vi "plc_registers.vi"() -> ()   [LabVIEW 2023]
panel:
  in  "Array":T1(array[cluster])=[{"Name"="Rotate_CMD", "Address"=0, "Data Type"=enum."Int", "Reg Type"=enum."Input"}, {"Name"="Termex_CMD", "Address"=1, "Data Type"=enum."Int", "Reg Type"=enum."Input"}, {"Name"="Mix_CMD", "Address"=2, "Data Type"=enum."Int", "Reg Type"=enum."Input"}, {"Name"="Rotate_SP_Angle_Init", "Address"=3, "Data Type"=enum."Int", "Reg Type"=enum."Input"}, {"Name"="Rotate_SP_Angle_End", "Address"=4, "Data Type"=enum."Int", "Reg Type"=enum."Input"}, {"Name"="Rotate_SP_Timeout", "Address"=5, "Data Type"=enum."Int", "Reg Type"=enum."Input"}, {"Name"="Rotate_SP_Speed", "Address"=6, "Data Type"=enum."Int", "Reg Type"=enum."Input"}, {"Name"="Reserved", "Address"=7, "Data Type"=enum."Int", "Reg Type"=enum."Input"}, {"Name"="T_SP", "Address"=8, "Data Type"=enum."Float", "Reg Type"=enum."Input"}, {"Name"="KP", "Address"=10, "Data Type"=enum."Float", "Reg Type"=enum."Input"}, {"Name"="TN", "Address"=12, "Data Type"=enum."Float", "Reg Type"=enum."Input"}, {"Name"="Mix_SP", "Address"=14, "Data Type"=enum."Int", "Reg Type"=enum."Input"}, {"Name"="Reserved", "Address"=15, "Data Type"=enum."Int", "Reg Type"=enum."Input"}, {"Name"="Reserved", "Address"=16, "Data Type"=enum."Int", "Reg Type"=enum."Input"}, {"Name"="Reserved", "Address"=17, "Data Type"=enum."Int", "Reg Type"=enum."Input"}, {"Name"="Reserved", "Address"=18, "Data Type"=enum."Int", "Reg Type"=enum."Input"}]
  out "Output Map":T2(c390)
  out "Array 2":T1(array[cluster])=[{"Name"="Rotate_IND", "Address"=0, "Data Type"=enum."Int", "Reg Type"=enum."Input"}, {"Name"="Termex_IND", "Address"=1, "Data Type"=enum."Int", "Reg Type"=enum."Input"}, {"Name"="Mix_IND", "Address"=2, "Data Type"=enum."Int", "Reg Type"=enum."Input"}, {"Name"="Rotate_PV_Angle_Init", "Address"=3, "Data Type"=enum."Int", "Reg Type"=enum."Input"}, {"Name"="Rotate_PV_Angle_End", "Address"=4, "Data Type"=enum."Int", "Reg Type"=enum."Input"}, {"Name"="Rotate_PV_Timeout", "Address"=5, "Data Type"=enum."Int", "Reg Type"=enum."Input"}, {"Name"="Rotate_PV_Speed", "Address"=6, "Data Type"=enum."Int", "Reg Type"=enum."Input"}, {"Name"="Rotate_PV_Time", "Address"=7, "Data Type"=enum."Int", "Reg Type"=enum."Input"}, {"Name"="Rotate_PV_Angle", "Address"=8, "Data Type"=enum."Int", "Reg Type"=enum."Input"}, {"Name"="Termex_PV_In", "Address"=9, "Data Type"=enum."Float", "Reg Type"=enum."Input"}, {"Name"="Termex_PV_Out", "Address"=11, "Data Type"=enum."Float", "Reg Type"=enum."Input"}, {"Name"="Termex_SP", "Address"=13, "Data Type"=enum."Float", "Reg Type"=enum."Input"}, {"Name"="Termex_KP", "Address"=15, "Data Type"=enum."Float", "Reg Type"=enum."Input"}, {"Name"="Termex_TN", "Address"=17, "Data Type"=enum."Float", "Reg Type"=enum."Input"}, {"Name"="MIX_PV", "Address"=19, "Data Type"=enum."Int", "Reg Type"=enum."Input"}, {"Name"="P_PV", "Address"=20, "Data Type"=enum."Float", "Reg Type"=enum."Input"}, {"Name"="MM_PV", "Address"=22, "Data Type"=enum."Float", "Reg Type"=enum."Input"}]
  out "IND":T3 {"Rotate_IND" items=["стоп", "Качалка Режим Авто", "Качалка Режим Ручной"]; "Termex_IND" items=["Термостат старт"=1, "Термостат стоп"=0]; "Mix_IND" items=["Мешалка движение вперёд"=1, "Мешалка движение назад"=2, "Мешалка стоп"=0]}
  in  "CMD":T4 {"Mix_CMD" items=["Мешалка движение вперёд"=1, "Мешалка движение назад"=2, "Мешалка стоп"=9]; "Termex_CMD" items=["Термостат старт"=1, "Термостат стоп"=9]; "Rotate_CMD" items=["Качалка Дом"=1, "Качалка Режим Авто - Старт"=2, "Качалка Режим Ручной - Старт"=3, "Качалка Стоп"=9]}
  in  "all rows":string[][](array[string])=[["Control", "Адрес", "CMD", "Комментарий", "", "Indication", "Адрес", "ÑMD", "Комментарий"], ["Rotate_CMD", "0", "1", "(*Качалка Дом*)", "", "Rotate_IND", "0", "0", "стоп"], ["", "0", "2", "(*Качалка Режим Авто - Старт*)", "", "", "0", "1", "(*Качалка Режим Авто*)"], ["", "0", "3", "(*Качалка Режим Ручной - Старт*)", "", "", "0", "2", "(*Качалка Режим Ручной*)"], ["", "0", "9", "(*Качалка Стоп*)", "", "", "", "", ""], ["Termex_CMD", "1", "1", "(*Термостат старт*)", "", "Termex_IND", "1", "1", "(*Термостат старт*)"], ["", "1", "9", "(*Термостат стоп*)", "", "", "1", "0", "(*Термостат стоп*)"], ["Mix_CMD", "2", "1", "(*Мешалка движение вперёд*)", "", "Mix_IND", "2", "1", "(*Мешалка движение вперёд*)"], ["", "2", "2", "(*Мешалка движение назад*)", "", "", "2", "2", "(*Мешалка движение назад*)"], ["", "2", "9", "(*Мешалка стоп*)", "", "", "2", "0", "(*Мешалка стоп*)"], ["Rotate_SP_Angle_Init", "3", "", "(*Качалка начальный угол*)", "", "Rotate_PV_Angle_Init", "3", "", "(*Качалка заданный начальный угол*)"], ["Rotate_SP_Angle_End", "4", "", "(*Качалка конечный угол*)", "", "Rotate_PV_Angle_End", "4", "", "(*Качалка заданный конечный угол*)"], ["Rotate_SP_Timeout", "5", "", "(*Качалка время паузы*)", "", "Rotate_PV_Timeout", "5", "", "(*Качалка заданное время паузы*)"], ["Rotate_SP_Speed", "6", "", "(*Качалка скорость вращения*)", "", "Rotate_PV_Speed", "6", "", "(*Качалка заданная скорость вращения*)"], ["Reserved", "7", "", "", "", "Rotate_PV_Time", "7", "", "(*Качалка отсчитанное время паузы*)"], ["T_SP[0]", "8", "", "(*Термостат уставка 1 байт*)", "", "Rotate_PV_Angle", "8", "", "(*Качалка текущий угол*)"], ["T_SP[1]", "9", "", "(*Термостат уставка 2 байт*)", "", "Termex_PV_In[0]", "9", "", "(*Термостат текущая внутр. Т 1 байт*)"], ["KP[0]", "10", "", "(*Термостат КР 1 байт*)", "", "Termex_PV_In[1]", "10", "", "(*Термостат текущая внутр. Т 2 байт*)"], ["KP[1]", "11", "", "(*Термостат КР 2 байт*)", "", "Termex_PV_Out[0]", "11", "", "(*Термостат текущая внеш. Т 1 байт*)"], ["TN[0]", "12", "", "(*Термостат TN 1 байт*)", "", "Termex_PV_Out[1]", "12", "", "(*Термостат текущая внеш. Т 2 байт*)"], ["TN[1]", "13", "", "(*Термостат TN 2 байт*)", "", "Termex_SP[0]", "13", "", "(*Термостат текущая уставка 1 байт*)"], ["Mix_SP", "14", "", "(*Мешалка задание*)", "", "Termex_SP[1]", "14", "", "(*Термостат текущая уставка 2 байт*)"], ["Reserved", "15", "", "", "", "Termex_KP[0]", "15", "", "(*Термостат текущий KP 1 байт*)"], ["Reserved", "16", "", "", "", "Termex_KP[1]", "16", "", "(*Термостат текущий KP 2 байт*)"], ["Reserved", "17", "", "", "", "Termex_TN[0]", "17", "", "(*Термостат текущий TN 1 байт*)"], ["Reserved", "18", "", "", "", "Termex_TN[1]", "18", "", "(*Термостат текущий TN 2 байт*)"], ["", "", "", "", "", "MIX_PV", "19", "", "(*Мешалка текущая скорость*)"], ["", "", "", "", "", "P_PV[0]", "20", "", "(*Давление 1 байт*)"], ["", "", "", "", "", "P_PV[1]", "21", "", "(*Давление 2 байт*)"], ["", "", "", "", "", "MM_PV[0]", "22", "", "(*Показания линейки 1 байт*)"], ["", "", "", "", "", "MM_PV[1]", "23", "", "(*Показания линейки 2 байт*)"], ["", "", "", "", "", "", "", "", ""], ["", "", "", "", "", "", "", "", ""], ["", "", "", "", "", "", "", "", ""], ["", "", "", "", "", "", "", "", ""], ["", "", "", "", "", "", "", "", ""], ["", "", "", "", "", "", "", "", ""], ["", "", "", "", "", "", "", "", ""], ["", "", "", "", "", "", "", "", ""], ["", "", "", "", "", "", "", "", ""], ["", "", "", "", "", "", "", "", ""], ["", "", "", "", "", "", "", "", ""], ["", "", "", "", "", "", "", "", ""], ["", "", "", "", "", "", "", "", ""], ["", "", "", "", "", "", "", "", ""]]
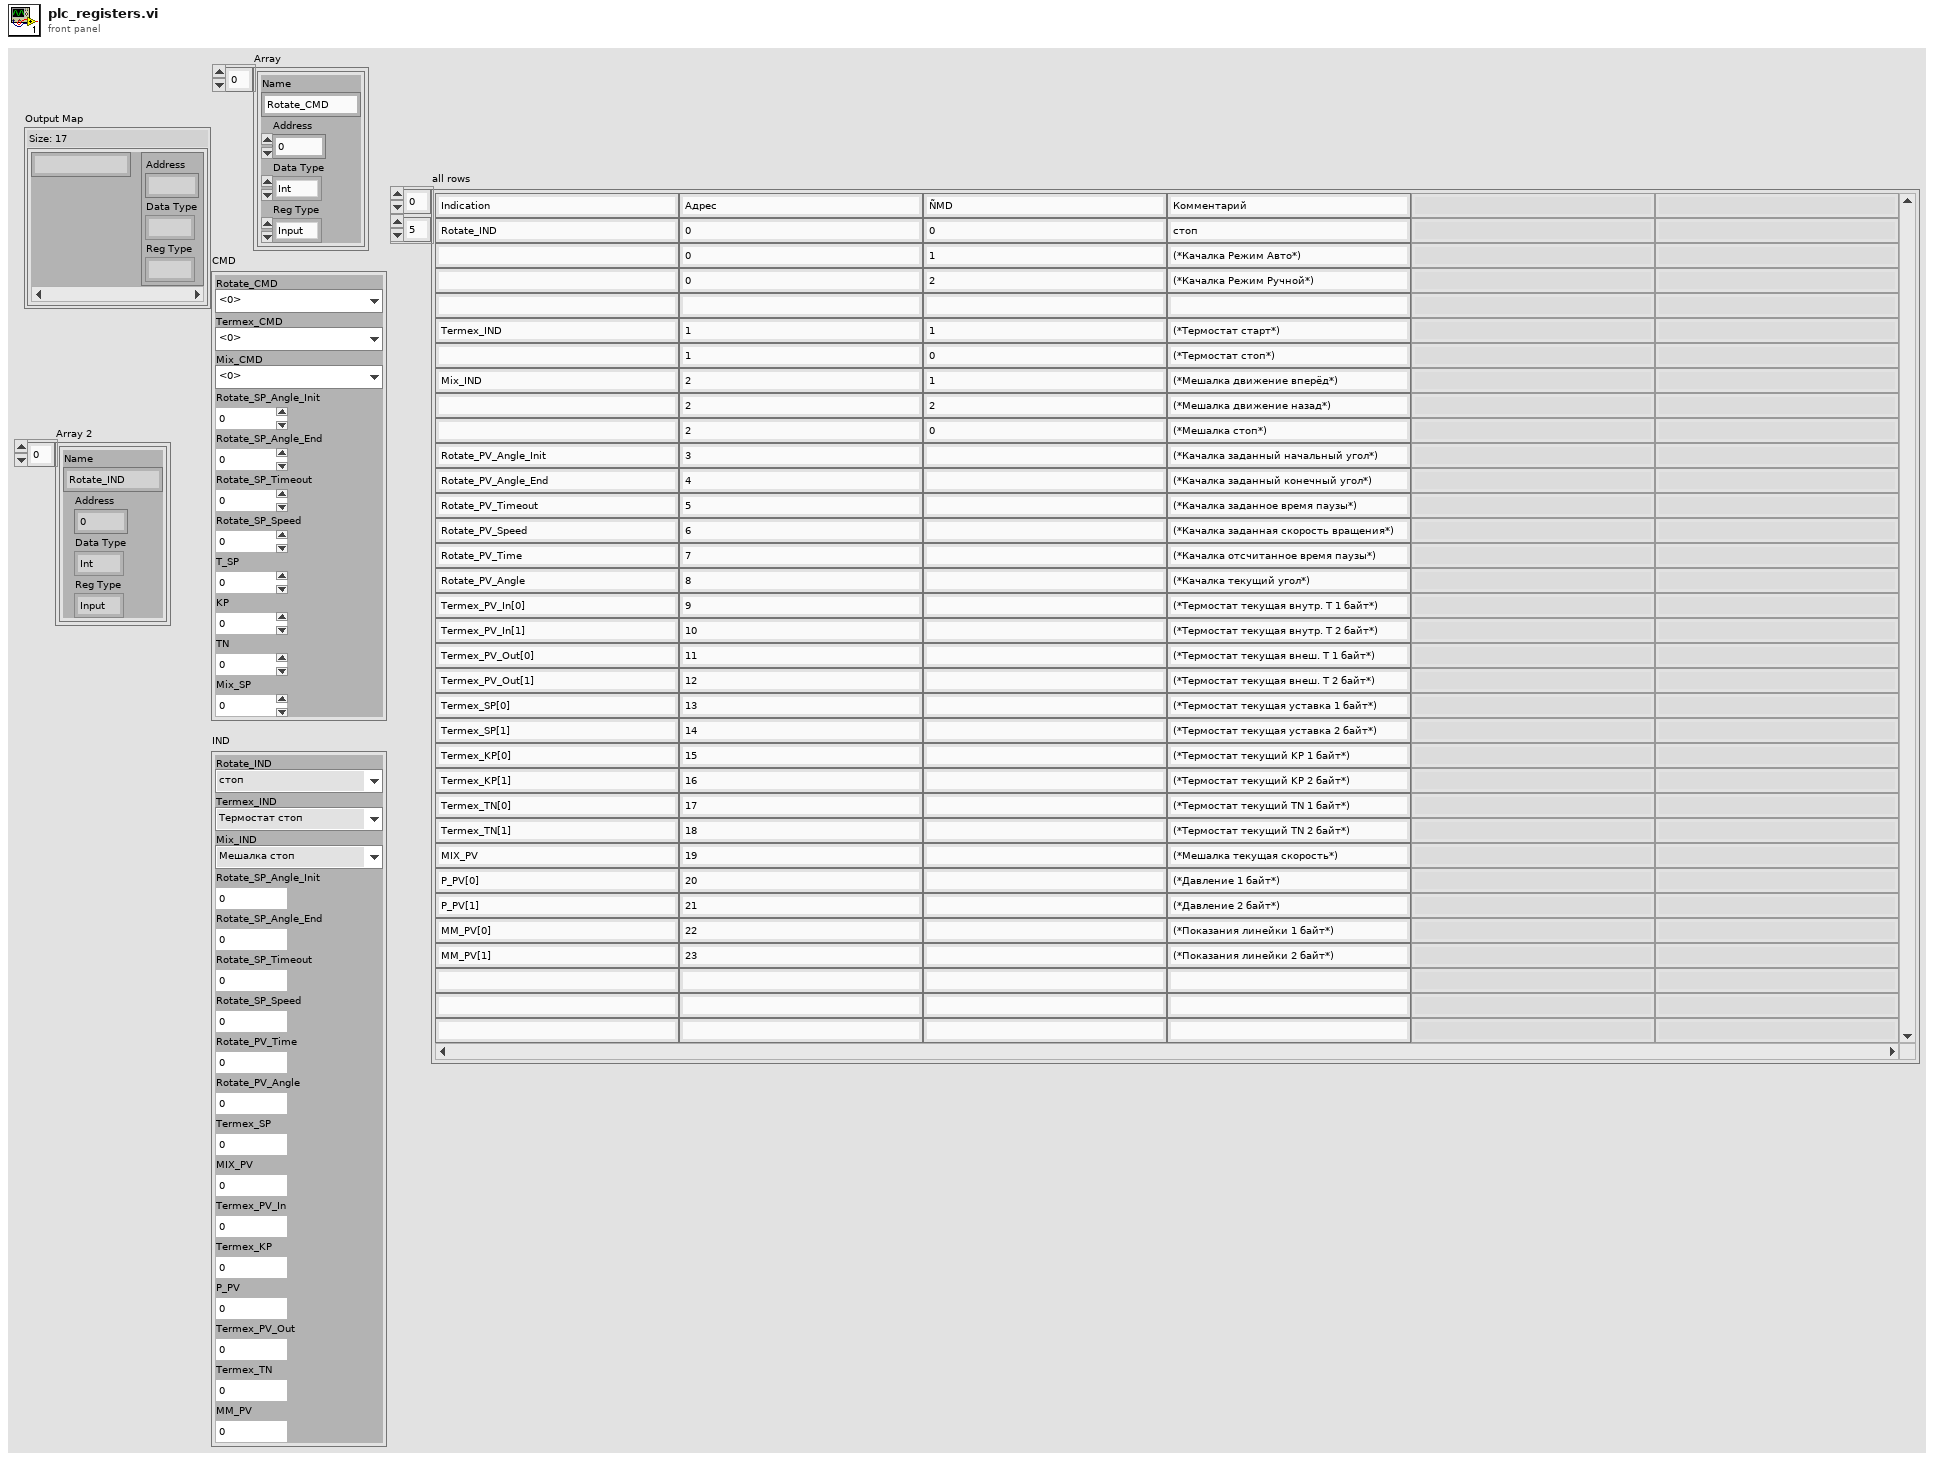
[diagram p1: front panel]
types:
  T1 = cluster{"Name":string, "Address":i32, "Data Type":enum16{"Int", "Float"}, "Reg Type":enum16{"Holding", "Input", "Coil"}}[]
  T2 = map{string, cluster{"Address":i32, "Data Type":enum16{"Int", "Float"}, "Reg Type":enum16{"Holding", "Input", "Coil"}}}
  T3 = cluster{"Rotate_IND":u16, "Termex_IND":u16, "Mix_IND":u16, "Rotate_SP_Angle_Init":u16, "Rotate_SP_Angle_End":u16, "Rotate_SP_Timeout":u16, "Rotate_SP_Speed":u16, "Rotate_PV_Time":u16, "Rotate_PV_Angle":u16, "Termex_SP":sgl, "MIX_PV":u16, "Termex_PV_In":sgl, "Termex_KP":sgl, "P_PV":sgl, "Termex_PV_Out":sgl, "Termex_TN":sgl, "MM_PV":sgl}
  T4 = cluster{"Rotate_CMD":u16, "Termex_CMD":u16, "Mix_CMD":u16, "Rotate_SP_Angle_Init":u16, "Rotate_SP_Angle_End":u16, "Rotate_SP_Timeout":u16, "Rotate_SP_Speed":u16, "T_SP":sgl, "KP":sgl, "TN":sgl, "Mix_SP":u16}
  T5 = cluster{"Name":string, "Address":i32, "Data Type":enum16{"Int", "Float"}, "Reg Type":enum16{"Holding", "Input", "Coil"}}
  T6 = cluster{"Address":i32, "Data Type":enum16{"Int", "Float"}, "Reg Type":enum16{"Holding", "Input", "Coil"}}
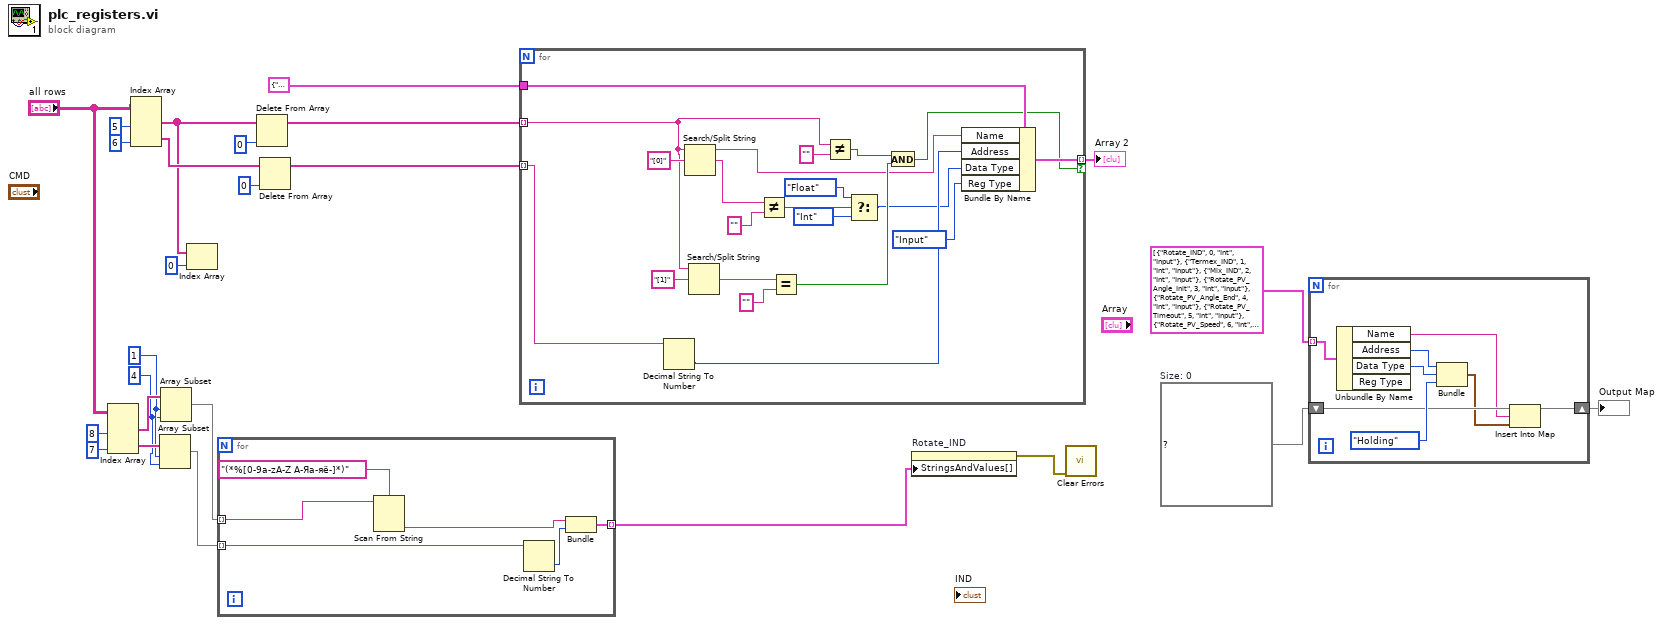
[diagram p0: block diagram]
diagram:
  w3 = T2 {}  # Size: 0
  w9 = 4 ("length")
  w10 = 1 ("index")
  n1 = Index Array(array="all rows", index (col) #1=8 ("disabled index (col)"), index (col) #2=7 ("index (col)")) -> (element #1=w12:string[], element #2=w11:string[])  [unwired: 2 in]
  n2 = Index Array(array="all rows", index (col) #1=5 ("disabled index (col)"), index (col) #2=6 ("index (col)")) -> (element #1=w15:string[], element #2=w22:string[])  [unwired: 2 in]
  n3 = Array Subset(array=w11, index=w10, length=w9) -> (w7:string[])
  n4 = Array Subset(array=w12, index=w10, length=w9) -> (w8:string[])
  n5 = Index Array(array=w15, index=0) -> ()  [unwired: 1 out]
  n6 = for {
    tunnel: w8 -> [w28] mode=indexing
    tunnel: w7 -> [w31] mode=indexing
    tunnel: [w30] -> w6 mode=indexing
    n7 = Scan From String(format string="(*%[0-9a-zA-Z А-Яа-яё-]*)", input string=w28) -> (output 1=w26:string)  [unwired: 3 in, 3 out]
    n8 = Decimal String To Number(string=w31) -> (number=w29:i32)  [unwired: 2 in, 1 out]
    n9 = Bundle(w26, w29) -> (w30:cluster{string, i32})  [unwired: 1 in]
  }
  n10 = Delete From Array(array=w15, index=0) -> (array with subset deleted=w20:string[])  [unwired: 1 in, 1 out]
  n11 = Delete From Array(array=w22, index=0) -> (array with subset deleted=w19:string[])  [unwired: 1 in, 1 out]
  n12 = for {
    tunnel: w20 -> [w32] mode=indexing
    tunnel: w19 -> [w37] mode=indexing
    tunnel: T5 {"Name"="", "Address"=0, "Data Type"=enum."Int", "Reg Type"=enum."Holding"} -> [w41]
    tunnel: [w40] -> w4 mode=indexing if=w39
    n13 = Decimal String To Number(string=w37) -> (number=w35:i32)  [unwired: 2 in, 1 out]
    n14 = Search/Split String(string=w32, search string/char (-)="[0]" ("input string")) -> (substring before match=w38:string, match + rest of string=w43:string)  [unwired: 1 in, 1 out]
    n15 = Search/Split String(string=w32, search string/char (-)="[1]" ("input string")) -> (match + rest of string=w44:string)  [unwired: 1 in, 2 out]
    n16 = Not Equal?(x=w43, y="") -> (x != y?=w49:bool)
    n17 = Equal?(x=w44, y="") -> (x = y?=w42:bool)
    n18 = Not Equal?(x=w32, y="") -> (x != y?=w46:bool)
    n19 = Select(t=enum16{"Int", "Float"}."Float", s=w49, f=enum16{"Int", "Float"}."Int") -> (s? t:f=w34:enum16{"Int", "Float"})
    n20 = And(x=w46, y=w42) -> (x .and. y?=w39:bool)
    n21 = Bundle By Name(cluster=w41, "Name"=w38, "Address"=w35, "Data Type"=w34, "Reg Type"=enum16{"Holding", "Input", "Coil"}."Input") -> (w40:T5)
  }
  "Array 2" <- w4
  n22 = property on="Rotate_IND" class="Ring (strict)"("StringsAndValues[]"=w6) -> (error out=w5:errorcluster)  [unwired: 2 in, 1 out]
  n23 = call <vilib>:"Clear Errors.vi"("error in (no error)"=w5) -> ()  [unwired: 5 in, 2 out]
  n24 = for {
    tunnel: T1 [{"Name"="Rotate_IND", "Address"=0, "Data Type"=enum."Int", "Reg Type"=enum."Input"}, {"Name"="Termex_IND", "Address"=1, "Data Type"=enum."Int", "Reg Type"=enum."Input"}, {"Name"="Mix_IND", "Address"=2, "Data Type"=enum."Int", "Reg Type"=enum."Input"}, {"Name"="Rotate_PV_Angle_Init", "Address"=3, "Data Type"=enum."Int", "Reg Type"=enum."Input"}, {"Name"="Rotate_PV_Angle_End", "Address"=4, "Data Type"=enum."Int", "Reg Type"=enum."Input"}, {"Name"="Rotate_PV_Timeout", "Address"=5, "Data Type"=enum."Int", "Reg Type"=enum."Input"}, {"Name"="Rotate_PV_Speed", "Address"=6, "Data Type"=enum."Int", "Reg Type"=enum."Input"}, {"Name"="Rotate_PV_Time", "Address"=7, "Data Type"=enum."Int", "Reg Type"=enum."Input"}, {"Name"="Rotate_PV_Angle", "Address"=8, "Data Type"=enum."Int", "Reg Type"=enum."Input"}, {"Name"="Termex_PV_In", "Address"=9, "Data Type"=enum."Float", "Reg Type"=enum."Input"}, {"Name"="Termex_PV_Out", "Address"=11, "Data Type"=enum."Float", "Reg Type"=enum."Input"}, {"Name"="Termex_SP", "Address"=13, "Data Type"=enum."Float", "Reg Type"=enum."Input"}, {"Name"="Termex_KP", "Address"=15, "Data Type"=enum."Float", "Reg Type"=enum."Input"}, {"Name"="Termex_TN", "Address"=17, "Data Type"=enum."Float", "Reg Type"=enum."Input"}, {"Name"="MIX_PV", "Address"=19, "Data Type"=enum."Int", "Reg Type"=enum."Input"}, {"Name"="P_PV", "Address"=20, "Data Type"=enum."Float", "Reg Type"=enum."Input"}, {"Name"="MM_PV", "Address"=22, "Data Type"=enum."Float", "Reg Type"=enum."Input"}] ("Array 2") -> [w60] mode=indexing
    shift-right: [w55] -> w2
    shift-left: w3 -> [w56]
    n25 = Unbundle By Name(w60) -> ("Name"=w54:string, "Address"=w59:i32, "Data Type"=w58:enum16{"Int", "Float"})  [unwired: 1 out]
    n26 = Bundle("Address"=w59, "Data Type"=w58, "Reg Type"=enum16{"Holding", "Input", "Coil"}."Holding") -> (w53:T6)  [unwired: 1 in]
    n27 = Insert Into Map(map in=w56, key=w54, value=w53) -> (map out=w55:T2)  [unwired: 2 out]
  }
  "Output Map" <- w2
